vi "Update Attributes.vi"(7 "Attributes in":refnum<class "Attributes.lvclass">, 9 "Transport":refnum<class "Transport.lvclass">, 10 "Actor Ref":refnum<vi>) -> (0 "Error out":errorcluster, 5 "Attributes out":refnum<class "Attributes.lvclass">)   [LabVIEW 2025, in "jettl.lvlib"]
uses:
  jettl.lvlib
  Attributes/Attributes.lvclass
  Transport/Transport.lvclass
  Attributes.ctl
  Msg Set.ctl
  Msg/Msg.lvclass
  Actor/Actor.lvclass
  Base Attributes/Base Attributes.lvlib
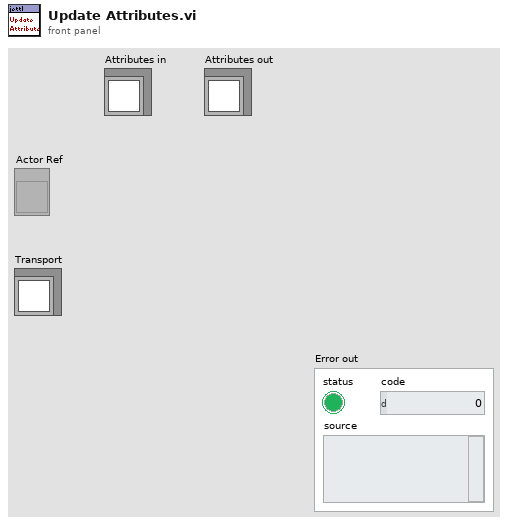
[diagram p1: front panel]
types:
  T1 = typedef "jettl.lvlib/Attributes.ctl" = cluster{"Unified Msg Set":T2, "UID":string, "Parent Attributes":refnum<class "Attributes.lvclass">, "Root":bool, "Persistent Layers":refnum<class "Actor.lvclass">[], "Application Ref":refnum<vi>, "Actor Ref":refnum<vi>, "Transport":refnum<class "Transport.lvclass">}
  T2 = typedef "jettl.lvlib/Msg Set.ctl" = set{refnum<class "Msg.lvclass">}
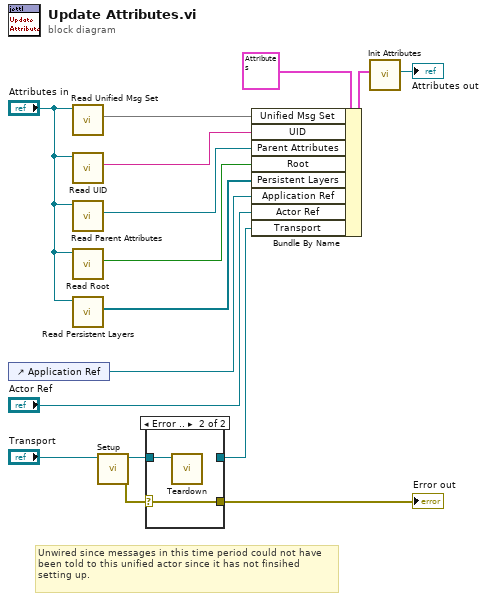
[diagram p0: block diagram]
diagram:
  # "Unwired since messages in this time period could not have been told to this unified actor since it has not finsihed setting up."
  n1 = control-ref of="Application Ref"() -> (w6:refnum<vi>)
  n2 = call-dynamic "Read Unified Msg Set.vi"("Attributes in"="Attributes in") -> ("Unified Msg Set"=w5:T2)  [unwired: 10 in]
  n3 = call-dynamic "Read UID.vi"("Attributes in"="Attributes in") -> ("UID"=w4:string)  [unwired: 10 in]
  n4 = call-dynamic "Read Parent Attributes.vi"("Attributes in"="Attributes in") -> ("Parent Attributes"=w3:refnum<class "Attributes.lvclass">)  [unwired: 10 in]
  n5 = call-dynamic "Read Root.vi"("Attributes in"="Attributes in") -> ("Root"=w2:bool)  [unwired: 10 in]
  n6 = call-dynamic "Read Persistent Layers.vi"("Attributes in"="Attributes in") -> ("Persistent Layers"=w1:refnum<class "Actor.lvclass">[])  [unwired: 10 in]
  n7 = call-dynamic "Setup.vi"("Transport in"="Transport") -> ("Error out"=w10:errorcluster, "Transport out"=w9:refnum<class "Transport.lvclass">)  [unwired: 9 in]
  n8 = case shown="Error .." w10 {
    selector: w10 -> [_ w18]
    tunnel: w9 -> [w17 w19]
    tunnel: [_ w18] -> w11
    tunnel: [w17 _] -> w8
    frame No Error {
    }
    frame Error {
      n9 = call-dynamic "Teardown.vi"("Transport in"=w19) -> ()  [unwired: 10 in, 1 out]
    }
  }
  "Error out" <- w11
  n10 = Bundle By Name(cluster=T1 {"Unified Msg Set"={}, "UID"="", "Parent Attributes"=refnum, "Root"=FALSE, "Persistent Layers"=[], "Application Ref"=refnum, "Actor Ref"=refnum, "Transport"=refnum} ("Attributes"), "Unified Msg Set"=w5, "UID"=w4, "Parent Attributes"=w3, "Root"=w2, "Persistent Layers"=w1, "Application Ref"=w6, "Actor Ref"="Actor Ref", "Transport"=w8) -> (w14:T1)
  n11 = call "Init Attributes.vi"("Attributes"=w14) -> ("Attributes"=→"Attributes out":refnum<class "Attributes.lvclass">)  [unwired: 10 in]
